vi "Data Access.vi"(8 "error in (no error)":errorcluster, 10 "Data Access Handler":refnum<class "Data Access Handler.lvclass">, 11 "Reorder Driver Aliases Msg in":refnum<class "Reorder Driver Aliases Msg.lvclass">) -> (0 "error out":errorcluster, 3 "Reorder Driver Aliases Msg out":refnum<class "Reorder Driver Aliases Msg.lvclass">)   [LabVIEW 2020, in "Instrument Handler.lvlib" / "Reorder Driver Aliases Msg.lvclass"]
doc: "Expose class private data to the front panel while letting the Data Access Handler class act on the data."
uses:
  Reorder Driver Aliases Msg.lvclass
  C:/Current projects/WS/Framework/Framework/Actors/Instrument Handler/Instrument Handler Messages/Instrument Handler Response Msg/Instrument Handler Response Msg.lvclass
  C:/Current projects/WS/PPL/HDH.Actor Framework.Core.Msg.lvlibp/Flex Msg/Flex Msg.lvclass
  PPL/HDH.Actor Framework.Core.Msg.lvlibp/Flex Msg/Data Access Handlers/Data Access Handler/Data Access Handler.lvclass
  PPL/HDH.Actor Framework.Core.Publisher.lvlibp/Messages/Response Msg/Response Core/Controls/Ctl_SendFunction.ctl
  Instrument Handler Response Msg/Instrument Handler Response Msg.lvclass/Instrument Handler Response Msg.ctl
  Reorder Driver Aliases Msg.lvclass/Reorder Driver Aliases Msg.ctl
  PPL/HDH.Actor Framework.Core.Actor.lvlibp/1abvi3w/vi.lib/ActorFramework/Message Enqueuer/Message Priority.ctl
  Instrument Handler Response Msg/Instrument Handler Response Msg.lvclass
  PPL/HDH.Actor Framework.Core.Actor.lvlibp/1abvi3w/vi.lib/ActorFramework/Message Enqueuer/Message Enqueuer.lvclass
  PPL/HDH.Actor Framework.Core.Publisher.lvlibp
panel:
  in  "New indices":u32[](array[numeric])
  in  "Driver Name":string
  in  "Send Function(Await Reply)":T1=enum."Await Reply"
  in  "Timeout if Waiting(-1ms)":i32=-1
  in  "Cancel":bool
  in  "OK":bool
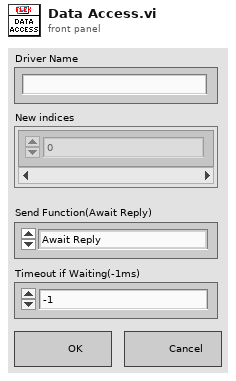
[diagram p1: front panel]
types:
  T1 = typedef "HDH.Actor Framework.Core.Publisher.lvlibp/Ctl_SendFunction.ctl" = enum16{"Send and Forget", "Request Reply", "Await Reply"}
  T2 = typedef "HDH.Actor Framework.Core.Actor.lvlibp/Message Enqueuer.lvclass/Message Priority.ctl" = enum16{"Low", "Normal", "High"}
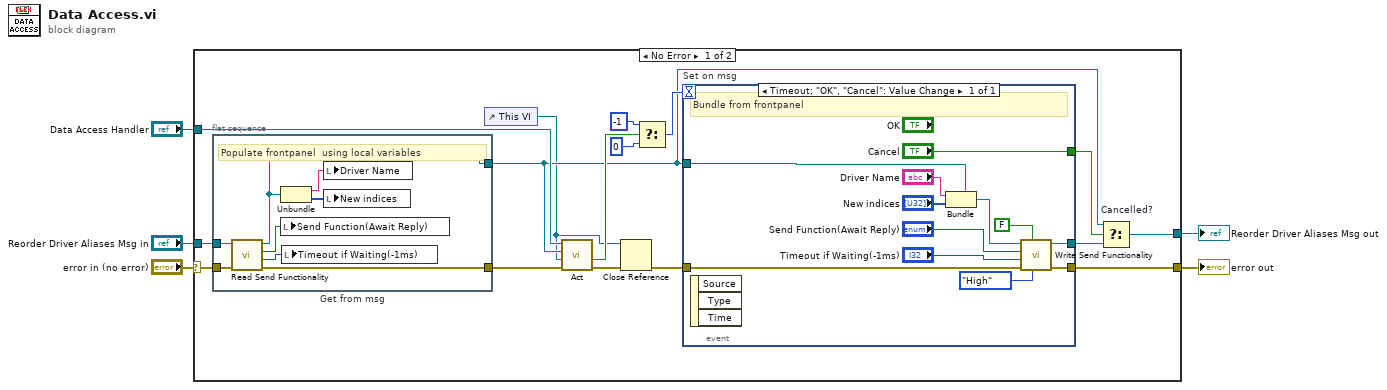
[diagram p0: block diagram]
diagram:
  n1 = case shown="No Error" "error in (no error)" {
    selector: "error in (no error)" -> [w21 w43]
    tunnel: [w14 w43] -> w4
    tunnel: [w9 w42] -> w2
    tunnel: "Reorder Driver Aliases Msg in" -> [w12 w42]
    tunnel: "Data Access Handler" -> [w20 _]
    frame No Error {
      n2 = flat-sequence "Get from msg" {
        tunnel: w21 -> [w41]
        tunnel: [w36] -> w7
        tunnel: w12 -> [w39]
        tunnel: [w40] -> w19
        frame #0 {
          # "Populate frontpanel  using local variables"
          n3 = call "Read Send Functionality.vi"("error in (no error)"=w41, "Instrument Handler Reponse Msg in"=w39) -> ("error out"=w40:errorcluster, "Timeout if Waiting"=w37:i32, "Send Function"=w38:T1, "Instrument Handler Reponse Msg out"=w36:refnum<class "Reorder Driver Aliases Msg.lvclass">)  [unwired: 4 in, 2 out]
          n4 = Unbundle(w36) -> (w34:string, w35:u32[])
          n5 = local write "Send Function(Await Reply)"(w38) -> ()
          n6 = local write "Timeout if Waiting(-1ms)"(w37) -> ()
          n7 = local write "Driver Name"(w34) -> ()
          n8 = local write "New indices"(w35) -> ()
        }
      }
      n9 = control-ref of="This VI"() -> (w6:refnum<vi>)
      n10 = call-dynamic "Act.vi"("error in (no error)"=w19, "VI Refnum in"=w6, "Flex Msg type"=w7, "Data Access Handler in"=w20) -> ("error out"=w11:errorcluster, "Await user action?"=w18:bool)  [unwired: 5 in, 1 out]
      n11 = Close Reference(reference=w6, error in (no error)=w11) -> (error out=w13:errorcluster)
      n12 = Select(t=-1, s=w18, f=0 ("t")) -> (s? t:f=w15:i32)
      n13 = event "Set on msg" shown="[0] Timeout;  \"OK\", \"Cancel\": Value Change" {
        selector: _ -> [_]
        dyn-events: _ -> [_]
        timeout: w15 -> [_]
        tunnel: [w31] -> w14
        tunnel: w13 -> [w33]
        tunnel: ["Cancel"] -> w10
        tunnel: [w29] -> w8
        tunnel: w7 -> [w30]
        event Timeout; "OK", "Cancel": Value Change {
          # "Bundle from frontpanel"
          n14 = event-data() -> ()  [unwired: 1 in, 3 out]
          n15 = Bundle(cluster=w30, "Driver Name", "New indices") -> (w25:refnum<class "Reorder Driver Aliases Msg.lvclass">)
          n16 = call "Write Send Functionality.vi"("Message Priority"=Message_Priority."High", "Publish Data?(T)"=FALSE, "error in (no error)"=w33, "Timeout if Waiting(-1ms)"="Timeout if Waiting(-1ms)", "Send Function(Await Reply)"="Send Function(Await Reply)", "Instrument Handler Reponse Msg in"=w25) -> ("error out"=w31:errorcluster, "Instrument Handler Reponse Msg out"=w29:refnum<class "Reorder Driver Aliases Msg.lvclass">)  [unwired: 4 in]
        }
      }
      n17 = Select "Cancelled?"(t=w7, s=w10, f=w8) -> (s? t:f=w9:refnum<class "Reorder Driver Aliases Msg.lvclass">)
    }
    frame Error {
    }
  }
  "error out" <- w4
  "Reorder Driver Aliases Msg out" <- w2
